vi "fg_Image Arrays.vi"(9 "Function":T2, 10 "Green Images Array in":T1[](array[typedef]), 11 "Red Images Array in":T1[](array[typedef])) -> (2 "Green Images Array":T1[](array[typedef]), 3 "Red Images Array":T1[](array[typedef]))   [LabVIEW 2017]
uses:
  Typedefs/Get-Set-Clear Control.ctl
  <vilib>/vision/Image Controls.llb/IMAQ Image.ctl
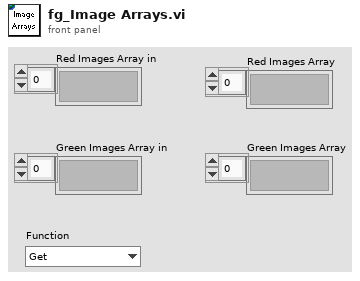
[diagram p1: front panel]
types:
  T1 = typedef "IMAQ Image.ctl" = refnum<image>
  T2 = typedef "Get-Set-Clear Control.ctl" = enum16{"Get", "Set", "Clear"}
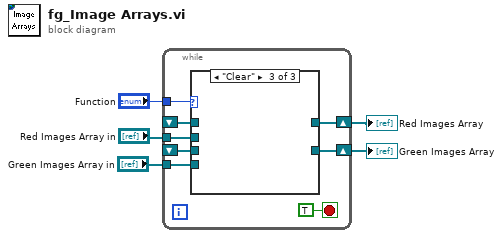
[diagram p0: block diagram]
diagram:
  n1 = while {
    shift-right: [w12] -> w4
    shift-left: _ -> [w10]
    tunnel: "Red Images Array in" -> [w11]
    tunnel: "Function" -> [w9]
    tunnel: "Green Images Array in" -> [w7]
    shift-right: [w8] -> w1
    shift-left: _ -> [w6]
    stop <- TRUE stop-if-true
    n2 = case shown="\"Clear\"" w9 {
      tunnel: [w15 w17 _] -> w12
      tunnel: w11 -> [_ w17 _]
      tunnel: w10 -> [w15 _ _]
      tunnel: [w14 w16 _] -> w8
      tunnel: w7 -> [_ w16 _]
      tunnel: w6 -> [w14 _ _]
      frame "Get", Default {
      }
      frame "Set" {
      }
      frame "Clear" {
      }
    }
  }
  "Red Images Array" <- w4
  "Green Images Array" <- w1
